vi "Configure Video Averaging.vi"(8 "error in (no error)":errorcluster, 9 "Video Averaging Count (4)":i32=4, 10 "Enable Video Averaging (F: Disable)":bool, 11 "VISA resource name":refnum<visa-resource-name>) -> (0 "error out":errorcluster, 3 "VISA resource name out":refnum<visa-resource-name>)   [LabVIEW 2014, in "Agilent U2000 Series.lvlib"]
doc: "Controls video averaging used to improve measurement accuracy.\n\nNote:\nFor 2040 X-Series, applicable for for U2042XA/U2044XA/U2049XA only."
uses:
  Agilent U2000 Series.lvlib
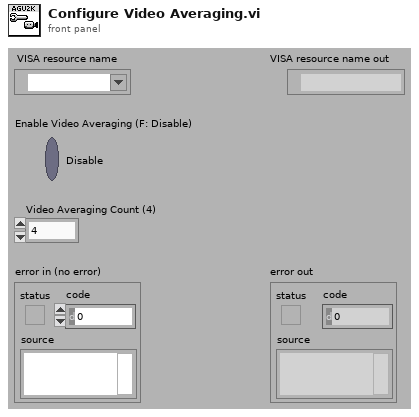
[diagram p1: front panel]
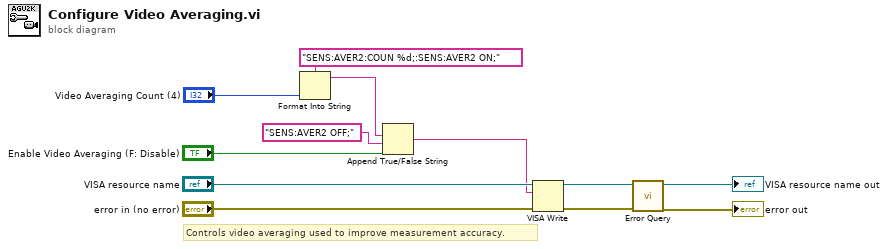
[diagram p0: block diagram]
diagram:
  # "Controls video averaging used to improve measurement accuracy."
  n1 = Format Into String(format string="SENS:AVER2:COUN %d;:SENS:AVER2 ON;", "Video Averaging Count (4)") -> (resulting string=w1:string)  [unwired: 2 in, 1 out]
  n2 = Append True/False String(1:"Enable Video Averaging (F: Disable)", 2:"SENS:AVER2 OFF;", 3:w1) -> (0:w2:string)  [unwired: 1 out]
  n3 = VISA Write(VISA resource name="VISA resource name", write buffer=w2, error in (no error)="error in (no error)") -> (VISA resource name out=w6:refnum<visa-resource-name>, error out=w5:errorcluster)  [unwired: 1 out]
  n4 = call "Error Query.vi"("error in (no error)"=w5, "VISA resource name"=w6) -> ("error out"=→"error out":errorcluster, "VISA resource name out"=→"VISA resource name out":refnum<visa-resource-name>)  [unwired: 8 out]
